vi "RTM - Remove Channels.vi"(8 "error in (no error)":errorcluster, 11 "Node Ptr In":T1 format="%.0x") -> (0 "error out":errorcluster)   [LabVIEW 2016, in "UDP-Custom-Device System Explorer.lvlib"]
uses:
  UDP-Custom-Device System Explorer.lvlib
  <vilib>/NI Veristand/Custom Device API/Custom Device Item Ref.ctl
  <vilib>/NI VeriStand/Custom Device Tools/Custom Device Utility Library/Custom Device Utility Library.lvlib
  <vilib>/NI VeriStand/Custom Device API/Custom Device API.lvlib
  Property Accessors/Tx Packet Accessors.lvlib
  Shared/UDP-Custom-Device Shared.lvlib
  Property Accessors/Shared Packet Accessors.lvlib
panel:
  in  "Tag":string
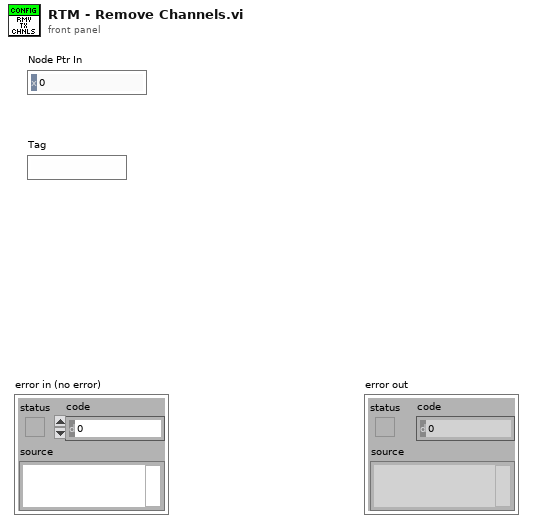
[diagram p1: front panel]
types:
  T1 = typedef "Custom Device API.lvlib/Custom Device Item Ref.ctl" = u64
  T2 = typedef "UDP-Custom-Device Shared.lvlib/Shared - Channel Data Type.ctl" = enum16{"Boolean", "Single", "Double", "I8", "I16", "I32", "I64", "U8", "U16", "U32", "U64"}
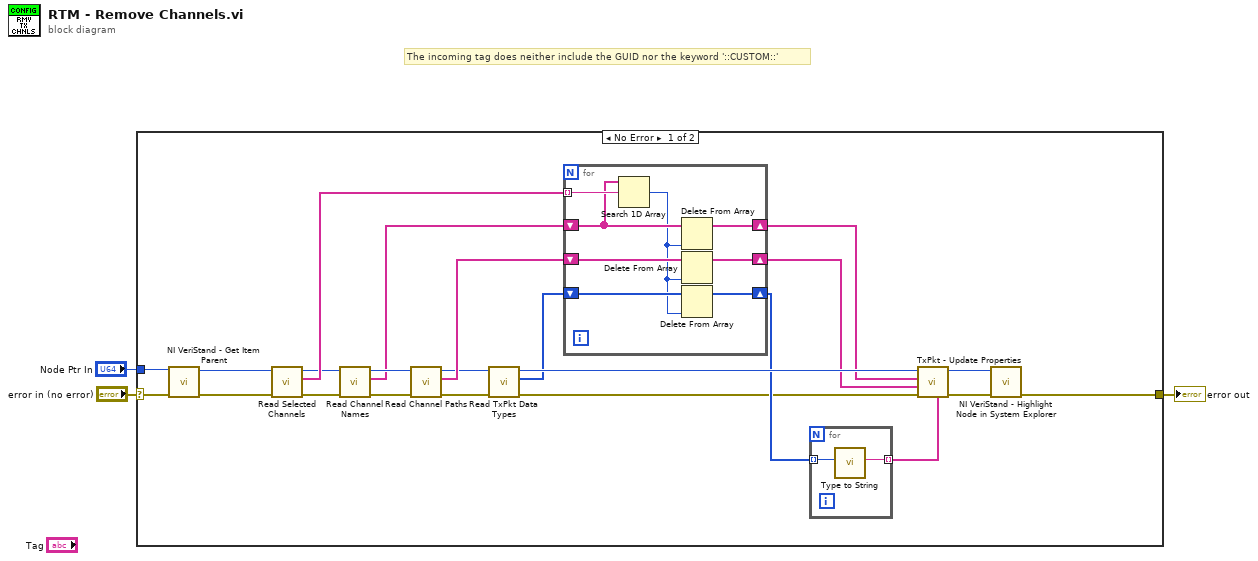
[diagram p0: block diagram]
diagram:
  # "The incoming tag does neither include the GUID nor the keyword '::CUSTOM::'"
  n1 = case shown="No Error" "error in (no error)" {
    selector: "error in (no error)" -> [w25 w37]
    tunnel: [w26 w37] -> w3
    tunnel: "Node Ptr In" -> [w24 _]
    frame No Error {
      n2 = call <vilib>:"NI VeriStand - Get Item Parent.vi"("error in (no error)"=w25, "Item Ref in"=w24) -> ("error out"=w9:errorcluster, "Item Ref out"=w14:T1)  [unwired: 6 in, 2 out]
      n3 = call "Read Selected Channels.vi"("error in (no error)"=w9, "Node Ptr"=w14) -> ("error out"=w10:errorcluster, "Selected Channel Names"=w13:string[], "Node Ptr out"=w12:T1)  [unwired: 7 in]
      n4 = call "Read Channel Names.vi"("error in (no error)"=w10, "Node Ptr"=w12) -> ("error out"=w8:errorcluster, "Channel Names"=w6:string[], "Node Ptr out"=w11:T1)  [unwired: 7 in]
      n5 = call "Read Channel Paths.vi"("error in (no error)"=w8, "Node Ptr"=w11) -> ("error out"=w4:errorcluster, "Channel Paths"=w7:string[], "Node Ptr out"=w5:T1)  [unwired: 7 in]
      n6 = call "Read TxPkt Data Types.vi"("error in (no error)"=w4, "Node Ptr"=w5) -> ("error out"=w19:errorcluster, "Data types"=w21:T2[], "Node Ptr out"=w22:T1)  [unwired: 7 in]
      n7 = for {
        tunnel: w13 -> [w34] mode=indexing
        shift-right: [w29] -> w17
        shift-left: w6 -> [w33]
        shift-right: [w30] -> w16
        shift-left: w7 -> [w36]
        shift-right: [w31] -> w20
        shift-left: w21 -> [w35]
        n8 = Search 1D Array(1D array=w33, element=w34) -> (index of element=w32:i32)  [unwired: 1 in]
        n9 = Delete From Array(array=w33, index=w32) -> (array with subset deleted=w29:string[])  [unwired: 1 in, 1 out]
        n10 = Delete From Array(array=w36, index=w32) -> (array with subset deleted=w30:string[])  [unwired: 1 in, 1 out]
        n11 = Delete From Array(array=w35, index=w32) -> (array with subset deleted=w31:T2[])  [unwired: 1 in, 1 out]
      }
      n12 = for {
        tunnel: w20 -> [w28] mode=indexing
        tunnel: [w27] -> w18 mode=indexing
        n13 = call "Type to String.vi"("Data Type"=w28) -> ("String Type"=w27:string)  [unwired: 10 in]
      }
      n14 = call "TxPkt - Update Properties.vi"("Channel Data Types"=w18, "error in (no error)"=w19, "Channel Paths"=w16, "Channel Names"=w17, "Item Ref in"=w22) -> ("error out"=w15:errorcluster, "Item Ref out"=w23:T1)  [unwired: 5 in]
      n15 = call <vilib>:"NI VeriStand - Highlight Node in System Explorer.vi"("error in (no error)"=w15, "Item Ref in"=w23) -> ("error out"=w26:errorcluster)  [unwired: 8 in, 1 out]
    }
    frame Error {
    }
  }
  "error out" <- w3
